vi "3A PWM MotorControl FPGA.vi"() -> ()   [LabVIEW 2011]
uses:
  <vilib>/robotics/Utilities/FPGA Utilities/Generate Digital Pulse (uSec).vi
  <vilib>/robotics/Utilities/FPGA Utilities/NI_Robotics_FPGA Utilities.lvlib
panel:
  in  "SERVO 2 Duty in Ticks":u32
  in  "stop PWM":bool
  in  "SERVO 1 Duty in Ticks":u32
  # "Winch"
  # "Rudder"
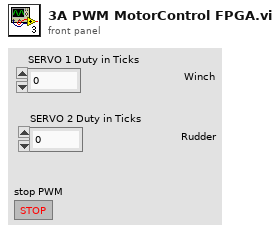
[diagram p1: front panel]
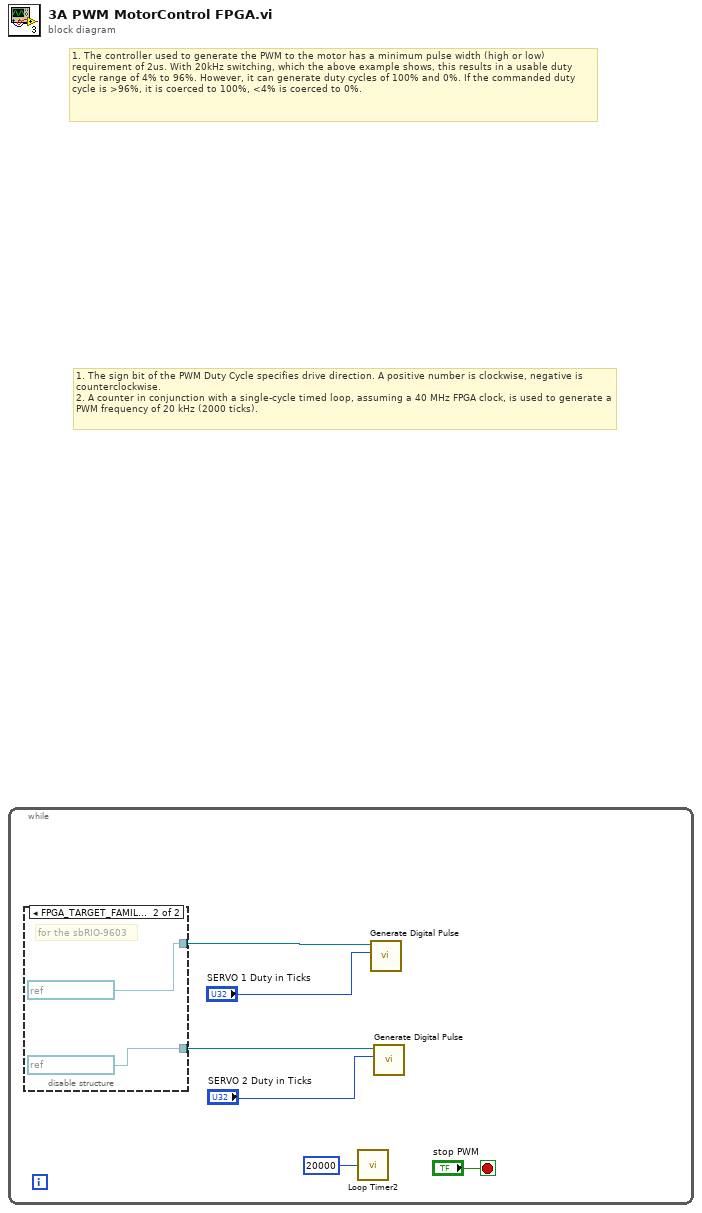
[diagram p0: block diagram]
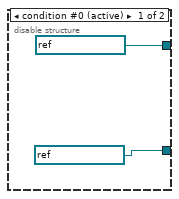
[diagram p2: hidden frame]
diagram:
  # "1. The sign bit of the PWM Duty Cycle specifies drive direction. A positive number is clockwise, negative is counterclockwise.\n2. A counter in conjunction with a single-cycle timed loop, assuming a 40 MHz FPGA clock, is used to generate a PWM frequency of 20 kHz (2000 ticks)."
  # "1. The controller used to generate the PWM to the motor has a minimum pulse width (high or low) requirement of 2us. With 20kHz switching, which the above example shows, this results in a usable duty cycle range of 4% to 96%. However, it can generate duty cycles of 100% and 0%. If the commanded duty cycle is >96%, it is coerced to 100%, <4% is coerced to 0%."
  n1 = while {
    stop <- "stop PWM" stop-if-true
    n2 = disable-structure shown="FPGA_TARGET_FAMILY==SPARTAN3" {
      disable-tunnel: [refnum<k21> "Mod4/DIO0" ("FPGA digital output") refnum<k21> "Port1/DIO1" ("Servo 1 digital output")] -> w2
      disable-tunnel: [refnum<k21> "Mod4/DIO1" ("FPGA digital output") refnum<k21> "Port0/DIO9" ("Servo 2 digital output 2")] -> w1
      frame condition #0 (active) {
      }
      frame condition #1 {
        # "for the sbRIO-9603"
      }
    }
    n3 = call "Loop Timer2"("Count(uSec)"=u32 20000) -> ()  [unwired: 1 out]
    n4 = call-poly <vilib>:"Generate Digital Pulse.vi"("pulse width (uSec)"="SERVO 1 Duty in Ticks", "FPGA digital output"=w2) -> ()  [unwired: 10 in]
    n5 = call-poly <vilib>:"Generate Digital Pulse.vi"("pulse width (uSec)"="SERVO 2 Duty in Ticks", "FPGA digital output"=w1) -> ()  [unwired: 10 in]
  }
